vi "Handle Request.vi"(7 "Processing In":refnum<class "Processing.lvclass">, 11 "Request Handler in":refnum<class "Request Handler.lvclass">) -> (0 "error out":errorcluster, 5 "Processing":refnum<class "Processing.lvclass">)   [LabVIEW 2020, in "HTTP Server.lvlib" / "Request Handler.lvclass"]
uses:
  Request Handler.lvclass
  Processing/Processing.lvclass
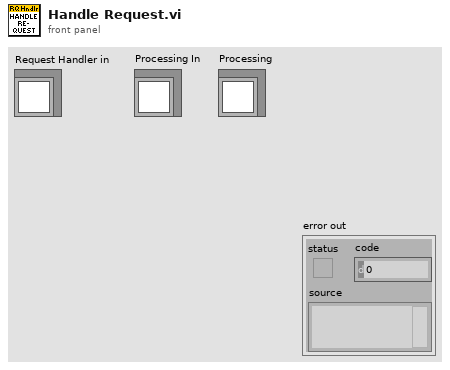
[diagram p1: front panel]
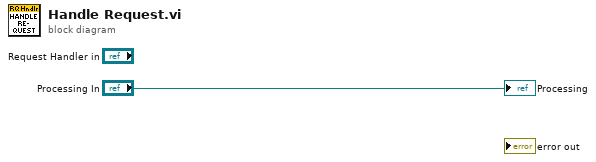
[diagram p0: block diagram]
diagram:
  "Processing" <- "Processing In"
